vi "Update Graphs_Brass.vi"(0 "Select Graph":T2, 2 "appended array":refnum<vi>[](array[refnum]), 5 "ERD Graph  Ind 2":T1, 11 "Error In":errorcluster) -> (12 "ERD 3":dbl(graph), 13 "ERD 2":dbl(graph), 14 "ERD 1":dbl(graph), 15 "Error Out":errorcluster)   [LabVIEW 2016]
doc: "This VI displays (makes visable) the corresponding graph based on user selection, as well as updates the values of the graphs with current data."
uses:
  type defs2/Select _Graph_Brass.ctl
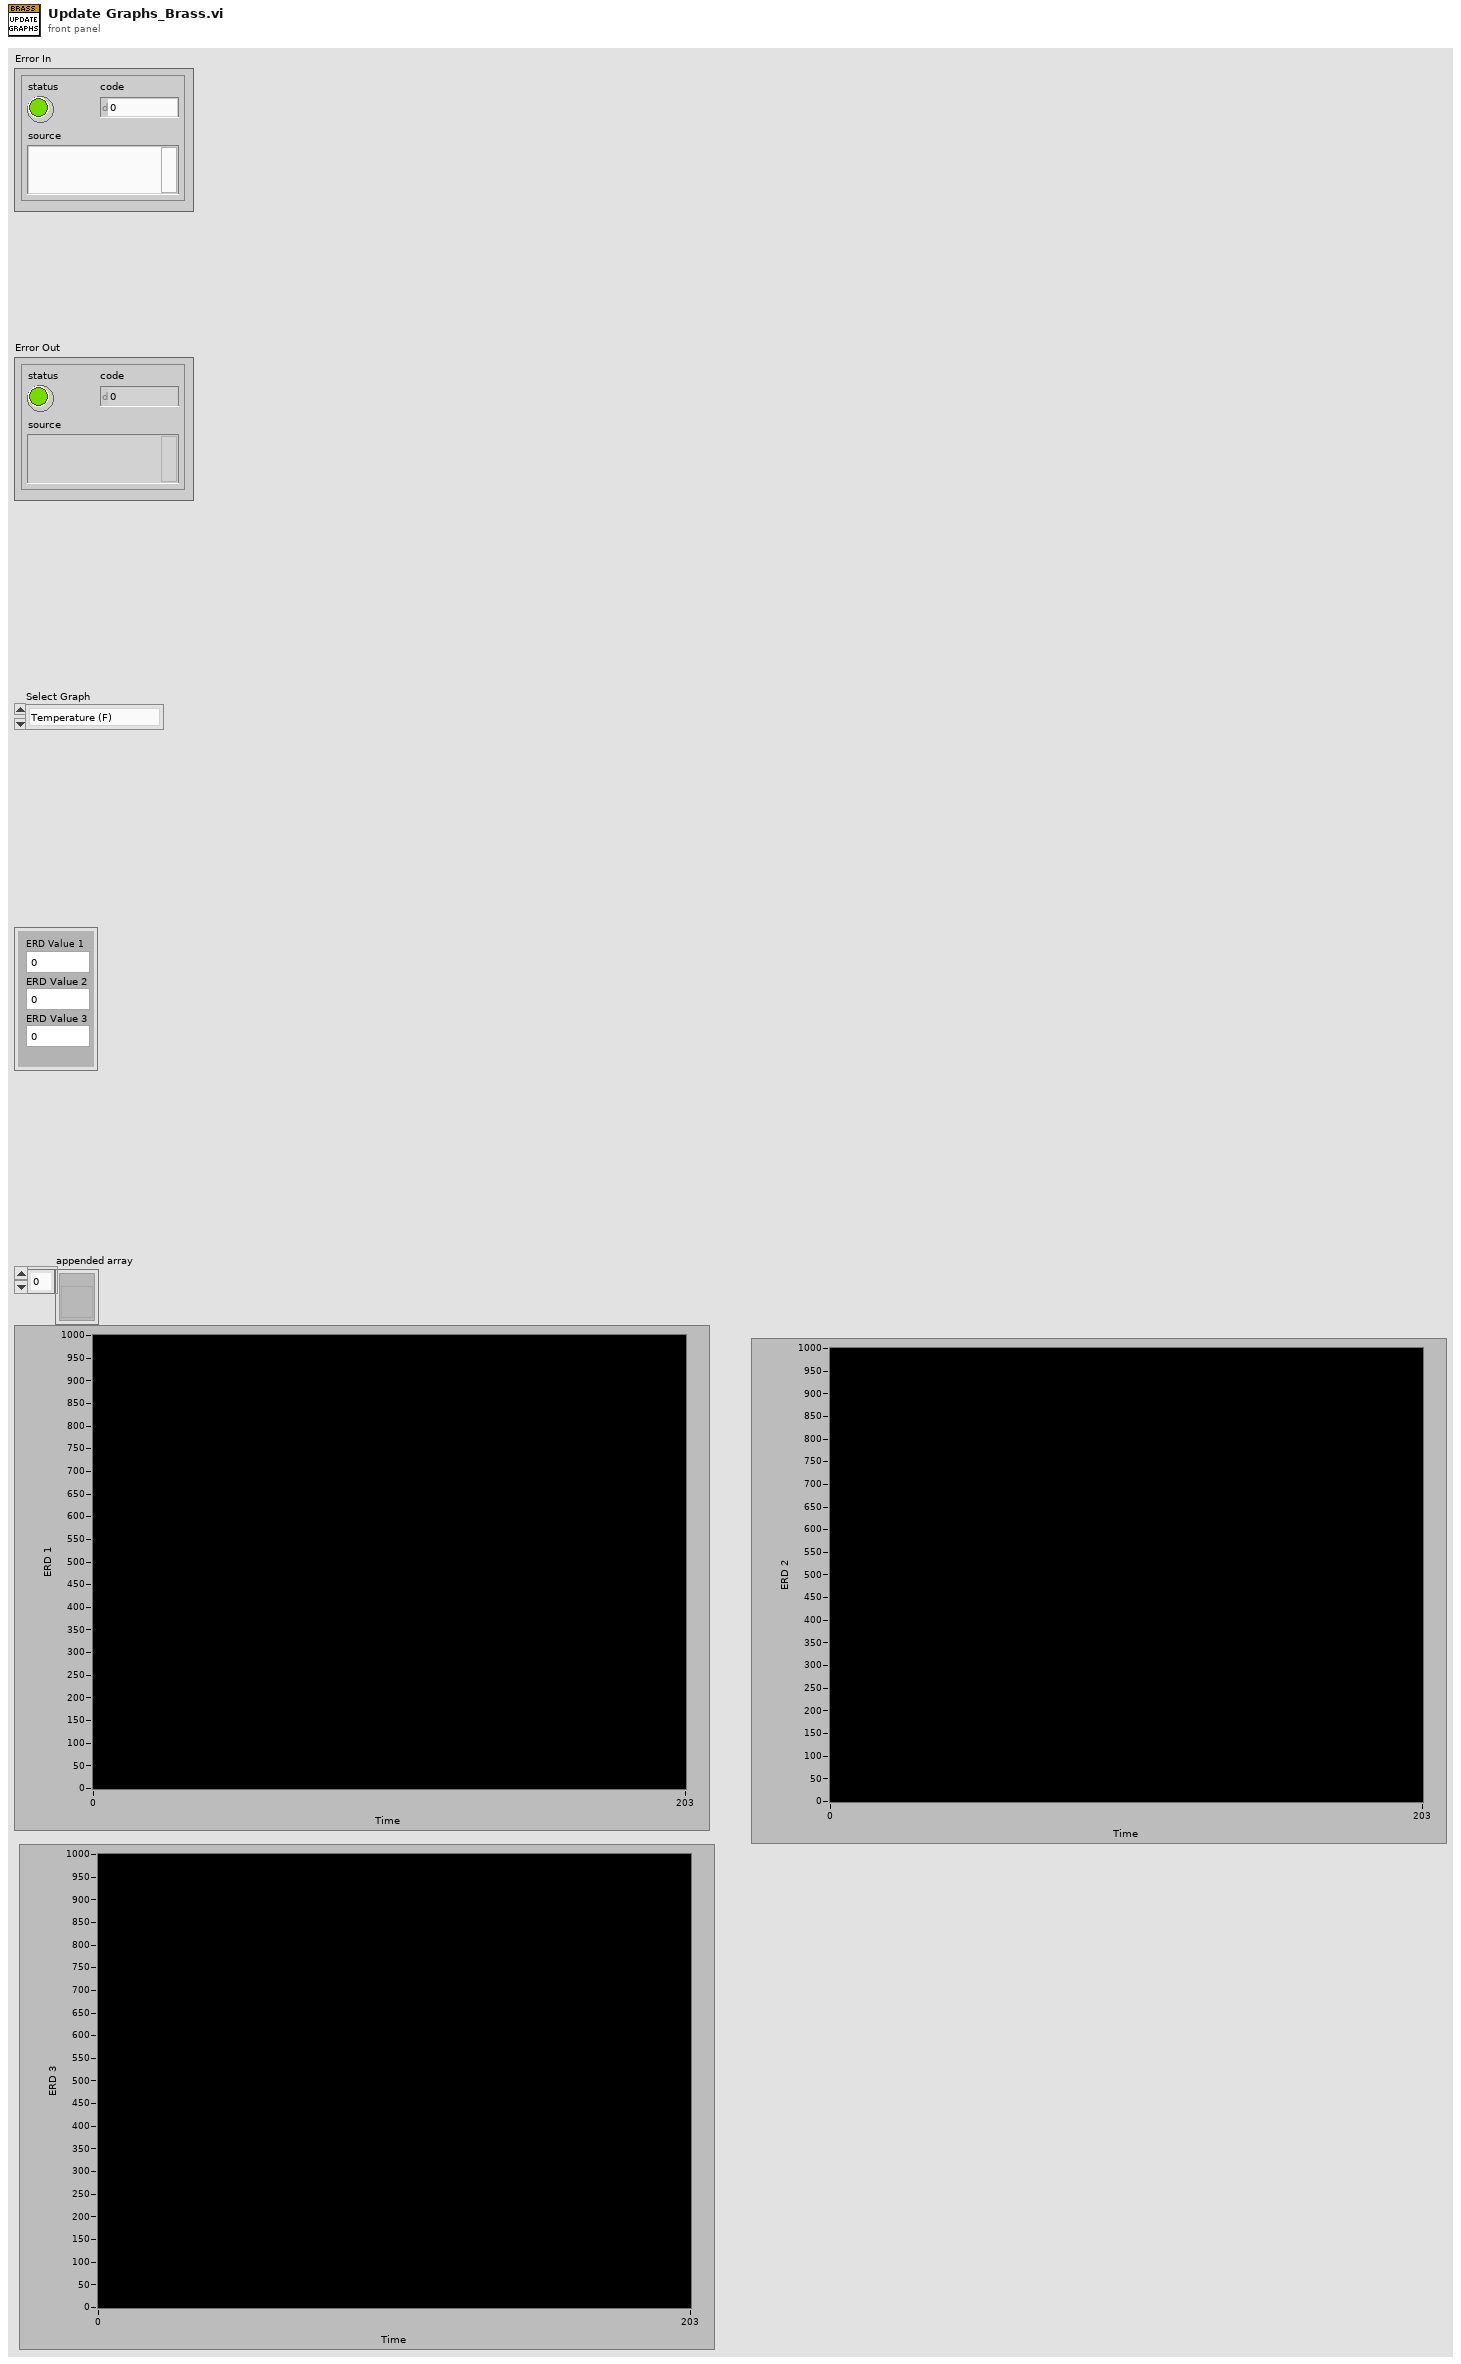
[diagram p1: front panel]
types:
  T1 = cluster{"ERD Value 1":dbl, "ERD Value 2":dbl, "ERD Value 3":dbl}
  T2 = typedef "Select _Graph_Brass.ctl" = enum16{"Temperature (F)", "Basket Speed (RPM)", "Tub Volume (Gal)", "Pressure (in H2O)", "Current RMS (Amps)", "ERD 1", "ERD 2", "ERD 3", "All Loads"}
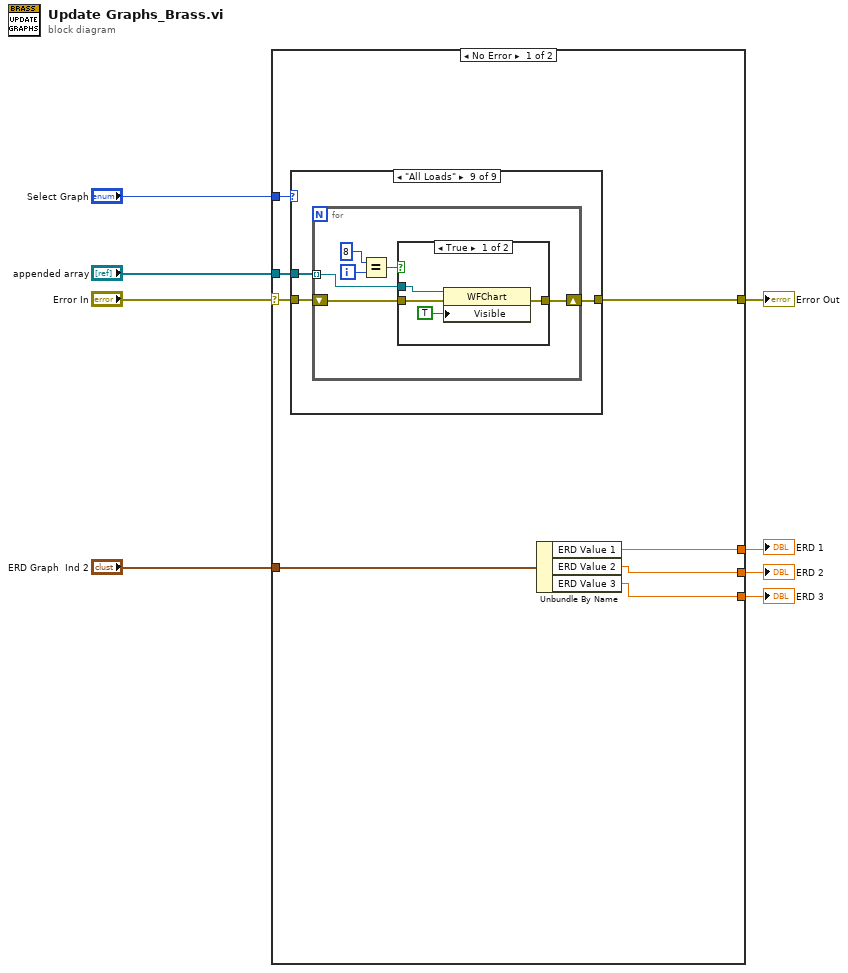
[diagram p0: block diagram]
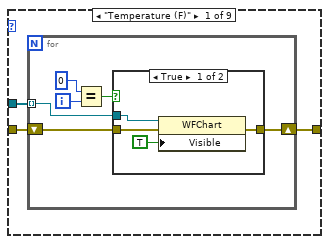
[diagram p2: hidden frame]
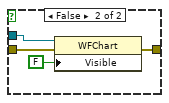
[diagram p3: hidden frame]
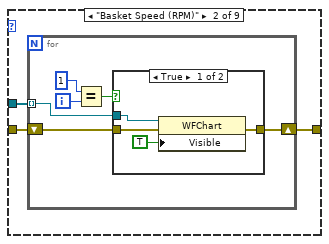
[diagram p4: hidden frame]
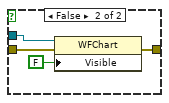
[diagram p5: hidden frame]
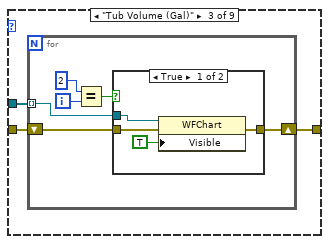
[diagram p6: hidden frame]
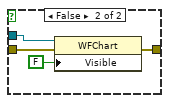
[diagram p7: hidden frame]
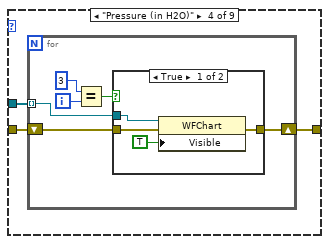
[diagram p8: hidden frame]
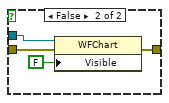
[diagram p9: hidden frame]
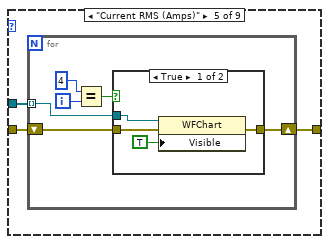
[diagram p10: hidden frame]
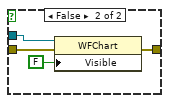
[diagram p11: hidden frame]
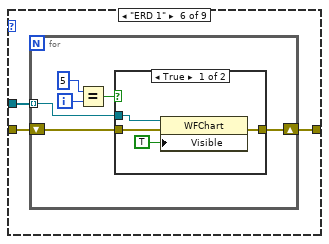
[diagram p12: hidden frame]
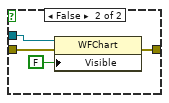
[diagram p13: hidden frame]
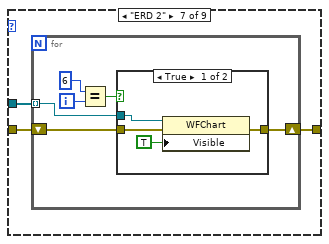
[diagram p14: hidden frame]
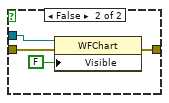
[diagram p15: hidden frame]
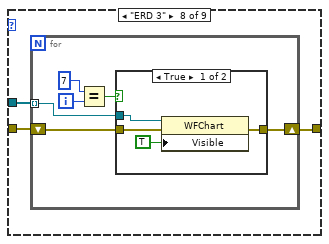
[diagram p16: hidden frame]
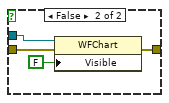
[diagram p17: hidden frame]
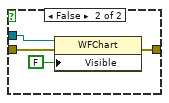
[diagram p18: hidden frame]
diagram:
  n1 = case shown="No Error" "Error In" {
    selector: "Error In" -> [w14 w170]
    tunnel: [w13 w170] -> w7
    tunnel: "appended array" -> [w15 _]
    tunnel: "Select Graph" -> [w16 _]
    tunnel: "ERD Graph  Ind 2" -> [w12 _]
    tunnel: [w11 _] -> w3
    tunnel: [w10 _] -> w2
    tunnel: [w9 _] -> w1
    frame No Error {
      n2 = case shown="\"All Loads\"" w16 {
        tunnel: w15 -> [w19 w36 w53 w70 w86 w103 w121 w136 w153]
        tunnel: w14 -> [w18 w35 w52 w69 w87 w104 w120 w138 w155]
        tunnel: [w17 w34 w51 w68 w85 w102 w119 w137 w154] -> w13
        frame "Temperature (F)" {
          n3 = for {
            tunnel: w19 -> [w25] mode=indexing
            shift-right: [w23] -> w17
            shift-left: w18 -> [w24]
            i -> [w22]
            n4 = Equal?(x=0 ("index"), y=w22) -> (x = y?=w20:bool)
            n5 = case shown="True" w20 {
              tunnel: w25 -> [w29 w33]
              tunnel: w24 -> [w27 w31]
              tunnel: [w26 w30] -> w23
              frame True {
                n6 = property class="WFChart"(reference=w29, error in=w27, "Visible"=TRUE) -> (error out=w26:errorcluster)  [unwired: 1 out]
              }
              frame False {
                n7 = property class="WFChart"(reference=w33, error in=w31, "Visible"=FALSE) -> (error out=w30:errorcluster)  [unwired: 1 out]
              }
            }
          }
        }
        frame "Basket Speed (RPM)" {
          n8 = for {
            tunnel: w36 -> [w42] mode=indexing
            shift-right: [w40] -> w34
            shift-left: w35 -> [w41]
            i -> [w39]
            n9 = Equal?(x=1 ("index"), y=w39) -> (x = y?=w37:bool)
            n10 = case shown="True" w37 {
              tunnel: w42 -> [w46 w50]
              tunnel: w41 -> [w44 w48]
              tunnel: [w43 w47] -> w40
              frame True {
                n11 = property class="WFChart"(reference=w46, error in=w44, "Visible"=TRUE) -> (error out=w43:errorcluster)  [unwired: 1 out]
              }
              frame False {
                n12 = property class="WFChart"(reference=w50, error in=w48, "Visible"=FALSE) -> (error out=w47:errorcluster)  [unwired: 1 out]
              }
            }
          }
        }
        frame "Tub Volume (Gal)" {
          n13 = for {
            tunnel: w53 -> [w59] mode=indexing
            shift-right: [w57] -> w51
            shift-left: w52 -> [w58]
            i -> [w56]
            n14 = Equal?(x=2 ("index"), y=w56) -> (x = y?=w54:bool)
            n15 = case shown="True" w54 {
              tunnel: w59 -> [w63 w67]
              tunnel: w58 -> [w61 w65]
              tunnel: [w60 w64] -> w57
              frame True {
                n16 = property class="WFChart"(reference=w63, error in=w61, "Visible"=TRUE) -> (error out=w60:errorcluster)  [unwired: 1 out]
              }
              frame False {
                n17 = property class="WFChart"(reference=w67, error in=w65, "Visible"=FALSE) -> (error out=w64:errorcluster)  [unwired: 1 out]
              }
            }
          }
        }
        frame "Pressure (in H2O)" {
          n18 = for {
            tunnel: w70 -> [w76] mode=indexing
            shift-right: [w74] -> w68
            shift-left: w69 -> [w75]
            i -> [w73]
            n19 = Equal?(x=3 ("index"), y=w73) -> (x = y?=w71:bool)
            n20 = case shown="True" w71 {
              tunnel: w76 -> [w80 w84]
              tunnel: w75 -> [w78 w82]
              tunnel: [w77 w81] -> w74
              frame True {
                n21 = property class="WFChart"(reference=w80, error in=w78, "Visible"=TRUE) -> (error out=w77:errorcluster)  [unwired: 1 out]
              }
              frame False {
                n22 = property class="WFChart"(reference=w84, error in=w82, "Visible"=FALSE) -> (error out=w81:errorcluster)  [unwired: 1 out]
              }
            }
          }
        }
        frame "Current RMS (Amps)" {
          n23 = for {
            tunnel: w86 -> [w93] mode=indexing
            shift-right: [w91] -> w85
            shift-left: w87 -> [w92]
            i -> [w90]
            n24 = Equal?(x=4 ("index"), y=w90) -> (x = y?=w88:bool)
            n25 = case shown="True" w88 {
              tunnel: w93 -> [w97 w101]
              tunnel: w92 -> [w95 w99]
              tunnel: [w94 w98] -> w91
              frame True {
                n26 = property class="WFChart"(reference=w97, error in=w95, "Visible"=TRUE) -> (error out=w94:errorcluster)  [unwired: 1 out]
              }
              frame False {
                n27 = property class="WFChart"(reference=w101, error in=w99, "Visible"=FALSE) -> (error out=w98:errorcluster)  [unwired: 1 out]
              }
            }
          }
        }
        frame "ERD 1" {
          n28 = for {
            tunnel: w103 -> [w110] mode=indexing
            shift-right: [w108] -> w102
            shift-left: w104 -> [w109]
            i -> [w107]
            n29 = Equal?(x=5 ("index"), y=w107) -> (x = y?=w105:bool)
            n30 = case shown="True" w105 {
              tunnel: w110 -> [w114 w118]
              tunnel: w109 -> [w112 w116]
              tunnel: [w111 w115] -> w108
              frame True {
                n31 = property class="WFChart"(reference=w114, error in=w112, "Visible"=TRUE) -> (error out=w111:errorcluster)  [unwired: 1 out]
              }
              frame False {
                n32 = property class="WFChart"(reference=w118, error in=w116, "Visible"=FALSE) -> (error out=w115:errorcluster)  [unwired: 1 out]
              }
            }
          }
        }
        frame "ERD 2" {
          n33 = for {
            tunnel: w121 -> [w127] mode=indexing
            shift-right: [w125] -> w119
            shift-left: w120 -> [w126]
            i -> [w124]
            n34 = Equal?(x=6 ("index"), y=w124) -> (x = y?=w122:bool)
            n35 = case shown="True" w122 {
              tunnel: w127 -> [w131 w135]
              tunnel: w126 -> [w129 w133]
              tunnel: [w128 w132] -> w125
              frame True {
                n36 = property class="WFChart"(reference=w131, error in=w129, "Visible"=TRUE) -> (error out=w128:errorcluster)  [unwired: 1 out]
              }
              frame False {
                n37 = property class="WFChart"(reference=w135, error in=w133, "Visible"=FALSE) -> (error out=w132:errorcluster)  [unwired: 1 out]
              }
            }
          }
        }
        frame "ERD 3" {
          n38 = for {
            tunnel: w136 -> [w144] mode=indexing
            shift-right: [w142] -> w137
            shift-left: w138 -> [w143]
            i -> [w141]
            n39 = Equal?(x=7 ("index"), y=w141) -> (x = y?=w139:bool)
            n40 = case shown="True" w139 {
              tunnel: w144 -> [w148 w152]
              tunnel: w143 -> [w146 w150]
              tunnel: [w145 w149] -> w142
              frame True {
                n41 = property class="WFChart"(reference=w148, error in=w146, "Visible"=TRUE) -> (error out=w145:errorcluster)  [unwired: 1 out]
              }
              frame False {
                n42 = property class="WFChart"(reference=w152, error in=w150, "Visible"=FALSE) -> (error out=w149:errorcluster)  [unwired: 1 out]
              }
            }
          }
        }
        frame "All Loads" {
          n43 = for {
            tunnel: w153 -> [w161] mode=indexing
            shift-right: [w159] -> w154
            shift-left: w155 -> [w160]
            i -> [w158]
            n44 = Equal?(x=8 ("index"), y=w158) -> (x = y?=w156:bool)
            n45 = case shown="True" w156 {
              tunnel: w161 -> [w165 w169]
              tunnel: w160 -> [w163 w167]
              tunnel: [w162 w166] -> w159
              frame True {
                n46 = property class="WFChart"(reference=w165, error in=w163, "Visible"=TRUE) -> (error out=w162:errorcluster)  [unwired: 1 out]
              }
              frame False {
                n47 = property class="WFChart"(reference=w169, error in=w167, "Visible"=FALSE) -> (error out=w166:errorcluster)  [unwired: 1 out]
              }
            }
          }
        }
      }
      n48 = Unbundle By Name(w12) -> ("ERD Value 1"=w11:dbl, "ERD Value 2"=w10:dbl, "ERD Value 3"=w9:dbl)
    }
    frame Error {
    }
  }
  "Error Out" <- w7
  "ERD 1" <- w3
  "ERD 2" <- w2
  "ERD 3" <- w1
